vi "Bark.vi"(8 "error in (no error)":errorcluster, 11 "Dog In":refnum<class "Dog.lvclass">) -> (0 "error out":errorcluster, 2 "Result":string, 3 "Dog Out":refnum<class "Dog.lvclass">)   [LabVIEW 2020, in "Dog.lvclass"]
uses:
  Dog.lvclass
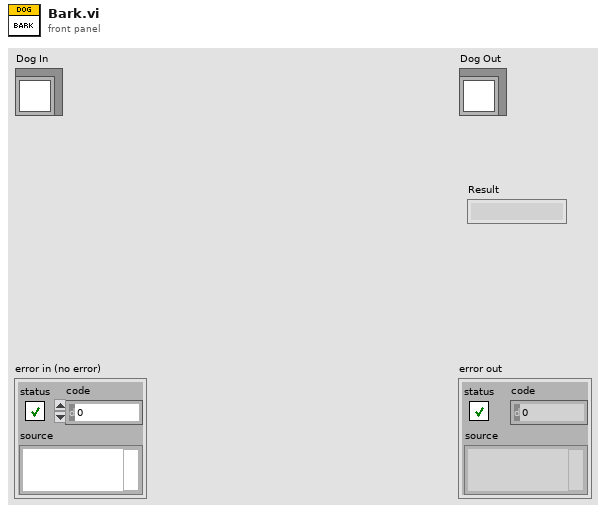
[diagram p1: front panel]
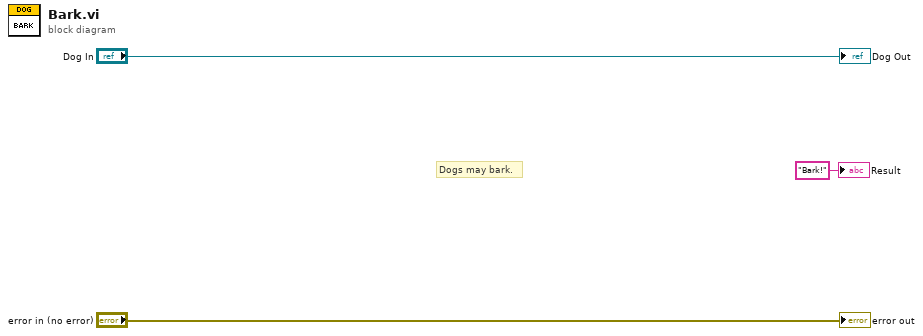
[diagram p0: block diagram]
diagram:
  # "Dogs may bark."
  "error out" <- "error in (no error)"
  "Dog Out" <- "Dog In"
  "Result" <- "Bark!" ("Result")
